vi "Measure.vi"(8 "error in (no error)":errorcluster, 9 "measurement configuration":variant, 10 "measure call context in":refnum<class "Measure Call Context.lvclass">, 11 "measurement plugin in":refnum<class "Automotive Ethernet Bus Monitor.lvclass">) -> (0 "error out":errorcluster, 1 "measurement results":variant, 2 "measure call context out":refnum<class "Measure Call Context.lvclass">, 3 "measurement plugin out":refnum<class "Automotive Ethernet Bus Monitor.lvclass">)   [LabVIEW 2025, in "Automotive Ethernet Bus Monitor.lvclass"]
uses:
  Automotive Ethernet Bus Monitor.lvclass
  <vilib>/Plug-In SDKs/Measurements/Measure Call Context/Measure Call Context.lvclass
  Measurement Configuration.ctl
  OOB gRPC Server/OOB gRPC Server.lvlib
  OOB Data Transfer/OOB Data Transfer.lvlib
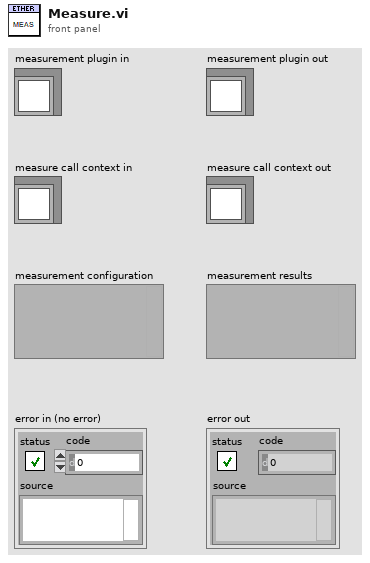
[diagram p1: front panel]
types:
  T1 = typedef "Automotive Ethernet Bus Monitor.lvclass/Measurement Configuration.ctl" = cluster{"CAPTURING STREAM":bool, "INTERFACE NAME STRING":string, "ETHERNET MODE IN":i32, "INTERFACE NAME":refnum<k21>}
  T2 = typedef "Automotive Ethernet Bus Monitor.lvclass/Measurement Results.ctl" = cluster{"Dataframe":string[][], "CAPTURING STREAM":bool, "RECEIVED PACKETS":i32, "OOB gRPC Port":i32, "STATUS":string}
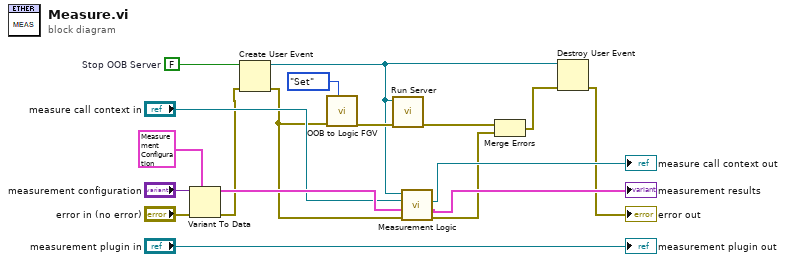
[diagram p0: block diagram]
diagram:
  w4 = FALSE  # Stop OOB Server
  n1 = Variant To Data(error in="error in (no error)", type=T1 {"CAPTURING STREAM"=TRUE, "INTERFACE NAME STRING"="", "ETHERNET MODE IN"=0, "INTERFACE NAME"="Lorem ipsum dolor sit"} ("measurement configuration"), Variant="measurement configuration") -> (data=w12:T1, error out=w3:errorcluster)
  n2 = Create User Event(user event datatype=w4, error in=w3) -> (user event=w1:refnum<user-event>, error out=w2:errorcluster)
  n3 = call "OOB to Logic FGV.vi"("Op (Get)"=enum16{"Get", "Set"}."Set", "error in (no error)"=w2) -> ("error out"=w10:errorcluster)  [unwired: 8 in, 1 out]
  n4 = call "Run Server.vi"("error in (no error)"=w10, "Stop OOB Server UE"=w1) -> ("error out"=w6:errorcluster)  [unwired: 9 in]
  n5 = call "Measurement Logic.vi"("error in"=w2, "measurement configuration"=w12, "measure call context in"="measure call context in", "Stop OOB Server UE"=w1) -> ("error out"=w5:errorcluster, "measurement results"=→"measurement results":T2, "measure call context out"=→"measure call context out":refnum<class "Measure Call Context.lvclass">)  [unwired: 5 in]
  n6 = Merge Errors(w6, w5) -> (w7:errorcluster)
  n7 = Destroy User Event(user event=w1, error in=w7) -> (error out=→"error out":errorcluster)
  "measurement plugin out" <- "measurement plugin in"
